vi "SwTmr Load Data.vi"(8 "error in (no error)":errorcluster) -> (0 "error out":errorcluster, 3 "New Graph Data":waveform(dbl)[](array[waveform]))   [LabVIEW 2017]
doc: "Loads data from a file on disk."
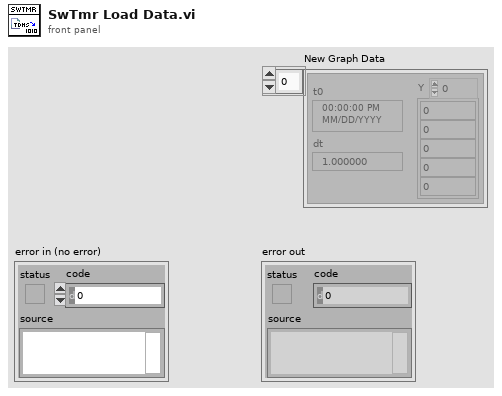
[diagram p1: front panel]
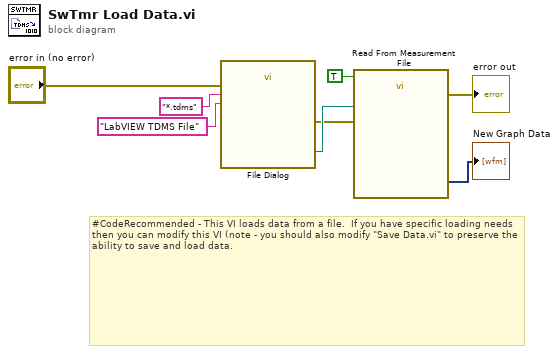
[diagram p0: block diagram]
diagram:
  # "#CodeRecommended - This VI loads data from a file.  If you have specific loading needs then you can modify this VI (note - you should also modify \"Save Data.vi\" to preserve the ability to save and load data."
  n1 = call "File Dialog"("error in"="error in (no error)", "pattern (all files)"="*.tdms", "pattern label"="LabVIEW TDMS File" ("LabVIEW TDMS File")) -> ("selected path"=w2:path, "error out"=w1:errorcluster)  [unwired: 9 in, 2 out]
  n2 = call "Read From Measurement File"("error in (no error)"=w1, "Filename"=w2, "Reset"=TRUE) -> ("error out"=→"error out":errorcluster, "Signals"=→"New Graph Data":dynamicdata)  [unwired: 3 in, 4 out]
